vi "Init Scan.vi"(8 "error in (no error)":errorcluster, 10 "Total Steps":u16, 11 "Cam_SLM_Controller in":refnum<class "Cam_SLM_Controller.lvclass">) -> (0 "error out":errorcluster, 3 "Cam_SLM_Controller out":refnum<class "Cam_SLM_Controller.lvclass">)   [LabVIEW 2023, in "Cam_SLM_controller.lvlib" / "Cam_SLM_Controller.lvclass"]
uses:
  Cam_SLM_Controller.lvclass
  Cam_SLM_Controller.lvclass/Cam_SLM_Controller.ctl
  Acq_comm_Interface Messages/External_Acq Msg/External_Acq Msg.lvclass
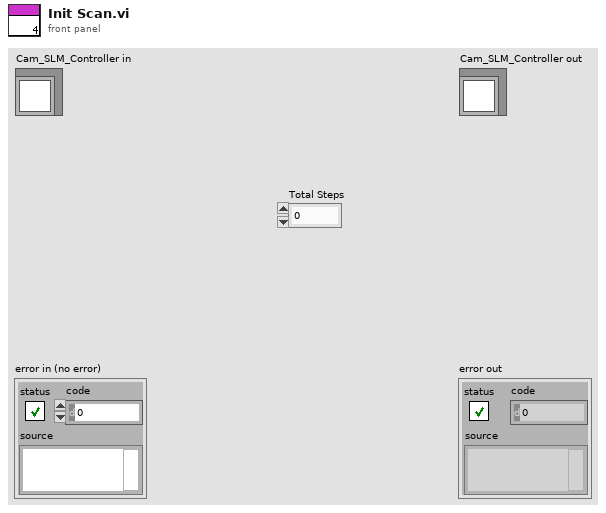
[diagram p1: front panel]
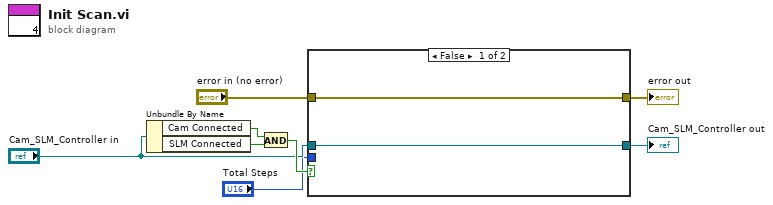
[diagram p0: block diagram]
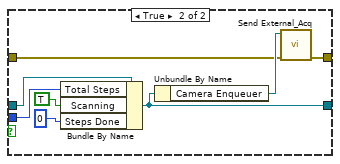
[diagram p2: hidden frame]
diagram:
  n1 = Unbundle By Name("Cam_SLM_Controller in") -> ("Cam Connected"=w8:bool, "SLM Connected"=w7:bool)
  n2 = And(x=w8, y=w7) -> (x .and. y?=w6:bool)
  n3 = case shown="False" w6 {
    tunnel: [w10 w15] -> w2
    tunnel: "Cam_SLM_Controller in" -> [w10 w18]
    tunnel: "Total Steps" -> [_ w13]
    tunnel: "error in (no error)" -> [w9 w12]
    tunnel: [w9 w11] -> w1
    frame False {
    }
    frame True {
      n4 = Bundle By Name(cluster=w18, "Total Steps"=w13, "Scanning"=TRUE, "Steps Done"=u16 0) -> (w15:refnum<class "Cam_SLM_Controller.lvclass">)
      n5 = Unbundle By Name(w15) -> ("Camera Enqueuer"=w14:refnum<class "Message Enqueuer.lvclass">)
      n6 = call "Send External_Acq.vi"("error in (no error)"=w12, "Message Enqueuer"=w14) -> ("error out"=w11:errorcluster)  [unwired: 8 in, 1 out]
    }
  }
  "error out" <- w1
  "Cam_SLM_Controller out" <- w2
